vi "Set Test Mode.vi"(8 "error in (no error)":errorcluster, 10 "Test Mode":enum16{"Tx", "Rx"}(ring), 11 "niDTS WLAN Dut Data in":refnum<class "niDTS WLAN Dut Data.lvclass">) -> (0 "error out":errorcluster, 3 "niDTS WLAN Dut Data out":refnum<class "niDTS WLAN Dut Data.lvclass">)   [LabVIEW 2015, in "niDTS WLAN.lvlib" / "niDTS WLAN Dut Data.lvclass"]
uses:
  niDTS WLAN Dut Data.lvclass
  niDTS WLAN Dut Data.lvclass/niDTS WLAN Dut Data.ctl
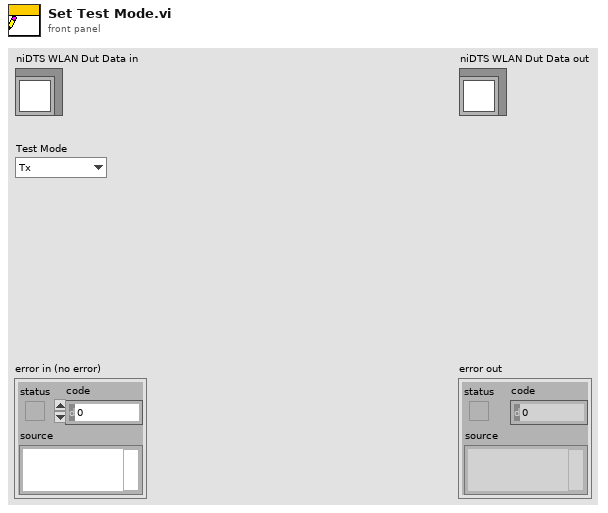
[diagram p1: front panel]
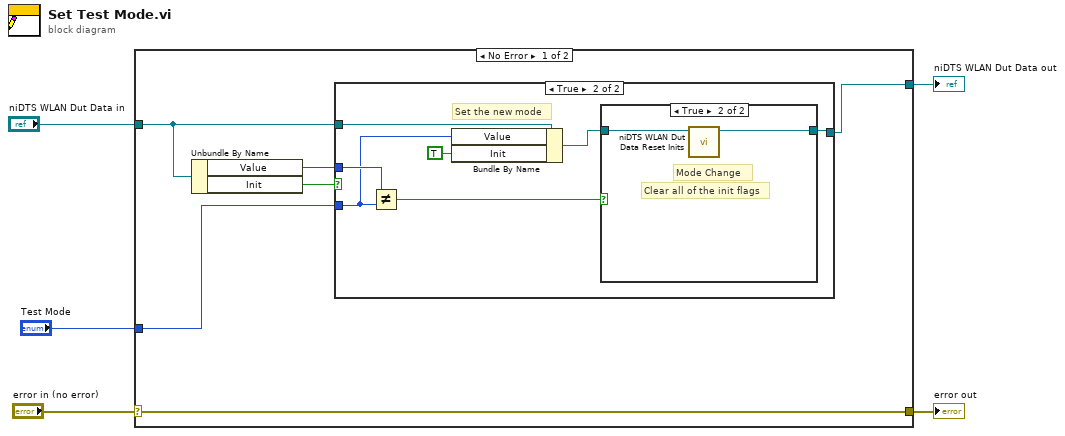
[diagram p0: block diagram]
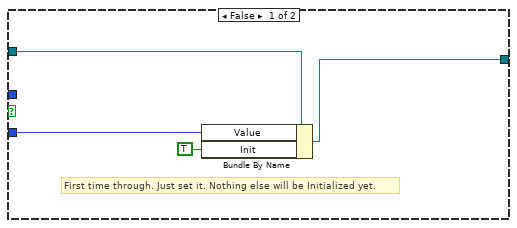
[diagram p2: hidden frame]
diagram:
  n1 = case shown="No Error" "error in (no error)" {
    selector: "error in (no error)" -> [w11 w26]
    tunnel: [w11 w26] -> w4
    tunnel: [w7 w27] -> w2
    tunnel: "niDTS WLAN Dut Data in" -> [w9 w27]
    tunnel: "Test Mode" -> [w8 _]
    frame No Error {
      n2 = Unbundle By Name(w9) -> ("Value"=w6:enum16{"Tx", "Rx"}, "Init"=w10:bool)
      n3 = case shown="True" w10 {
        tunnel: w9 -> [w15 w20]
        tunnel: w8 -> [w14 w19]
        tunnel: [w12 w16] -> w7
        tunnel: w6 -> [_ w22]
        frame False {
          # "First time through. Just set it. Nothing else will be Initialized yet."
          n4 = Bundle By Name(cluster=w15, "Value"=w14, "Init"=TRUE ("Test Mode.Init")) -> (w12:refnum<class "niDTS WLAN Dut Data.lvclass">)
        }
        frame True {
          # "Set the new mode"
          n5 = Not Equal?(x=w22, y=w19) -> (x != y?=w18:bool)
          n6 = Bundle By Name(cluster=w20, "Value"=w19, "Init"=TRUE ("Test Mode.Init")) -> (w17:refnum<class "niDTS WLAN Dut Data.lvclass">)
          n7 = case shown="True" w18 {
            tunnel: w17 -> [w23 w25]
            tunnel: [w23 w24] -> w16
            frame False {
              # "Equals. Mode is staying the same"
            }
            frame True {
              # "Clear all of the init flags"
              # "Mode Change"
              n8 = call-dynamic "niDTS WLAN Dut Data Reset Inits.vi"("niDTS WLAN Dut Data in"=w25) -> ("niDTS WLAN Dut Data out"=w24:refnum<class "niDTS WLAN Dut Data.lvclass">)  [unwired: 9 in, 1 out]
            }
          }
        }
      }
    }
    frame Error {
    }
  }
  "error out" <- w4
  "niDTS WLAN Dut Data out" <- w2
